vi "Traverse_Control_Ch_Names.vi"(1 "Traverse line":T1 {"Row Duration (mins)" format="%#.1f"; "Row No" min=0; "Trace Gas Concentration (%)" min=0.0 format="%#.2f"; "Emission Rate (l/min)" format="%#.2f"; "Tunnel Speed" format="%#.2f"; "Start X" format="%#.2f"; "Start Y" format="%#.2f"; "Start Z" format="%#.2f"; "End X" format="%#.2f"; "End Y" format="%#.2f"; "End Z" format="%#.2f"; "Averaging time (min)" min=0.0 format="%#.2f"}, 2 "Mode":T4(ring)) -> (0 "Channel names":string[](array[string]))   [LabVIEW 2013]
uses:
  Traverse_cluster.ctl
  Spacing.ctl
  Controls/Multi_run_mode.ctl
  Globals/Extra_Commands_Global.vi
panel:
  # "X           Y            Z"
  # "Start"
  # "End"
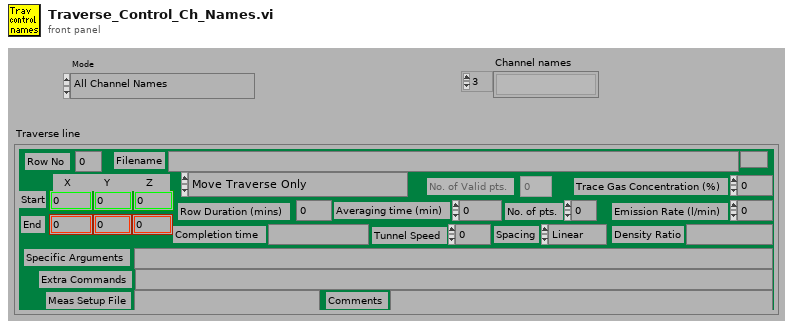
[diagram p1: front panel]
types:
  T1 = typedef "Traverse_cluster.ctl" = cluster{"Start X":dbl, "Start Y":dbl, "Start Z":dbl, "End X":dbl, "End Y":dbl, "End Z":dbl, "No. of pts.":i32, "Spacing":T2, "Filename":path, "Tunnel Speed":dbl, "Averaging time (min)":dbl, "Extra Commands":string, "Specific Arguments":string, "Emission Rate (l/min)":dbl, "Trace Gas Concentration (%)":dbl, "Density Ratio":string, "Comments":string, "Row No":i32, "Row Type Selector":T3, "Completion time":string, "Row Duration (mins)":dbl, "No. of Valid pts.":i32, "Meas Setup File":string}
  T2 = typedef "Spacing.ctl" = enum16{"Linear", "Log", "Gauss", "Specified", "N/A"}
  T3 = typedef "Multi_run_mode.ctl" = enum16{"Move Traverse Only", "Set Tunnel Speed Only", "Set Source Only", "Set Measurement Conditions", "Single Measurement", "Vertical Profile", "Lateral Profile", "Longitudinal Profile", "Explore Volume", "Multi-Axis Profile", "Auto Calibrate", "Meas Fast FID Bkgnd", "Check Beam Power", "Scanning Valve Measurement", "Run VI Named:", "Set ADAM Ch", "Wait (minutes)", "Send Message", "Synchronize With:", "Fall Back to this Row", "Turn Off Row Repeating", "Blank Row", "Traverse 3D Volume"}
  T4 = enum16{"All Channel Names", "Valid Channel Names"}
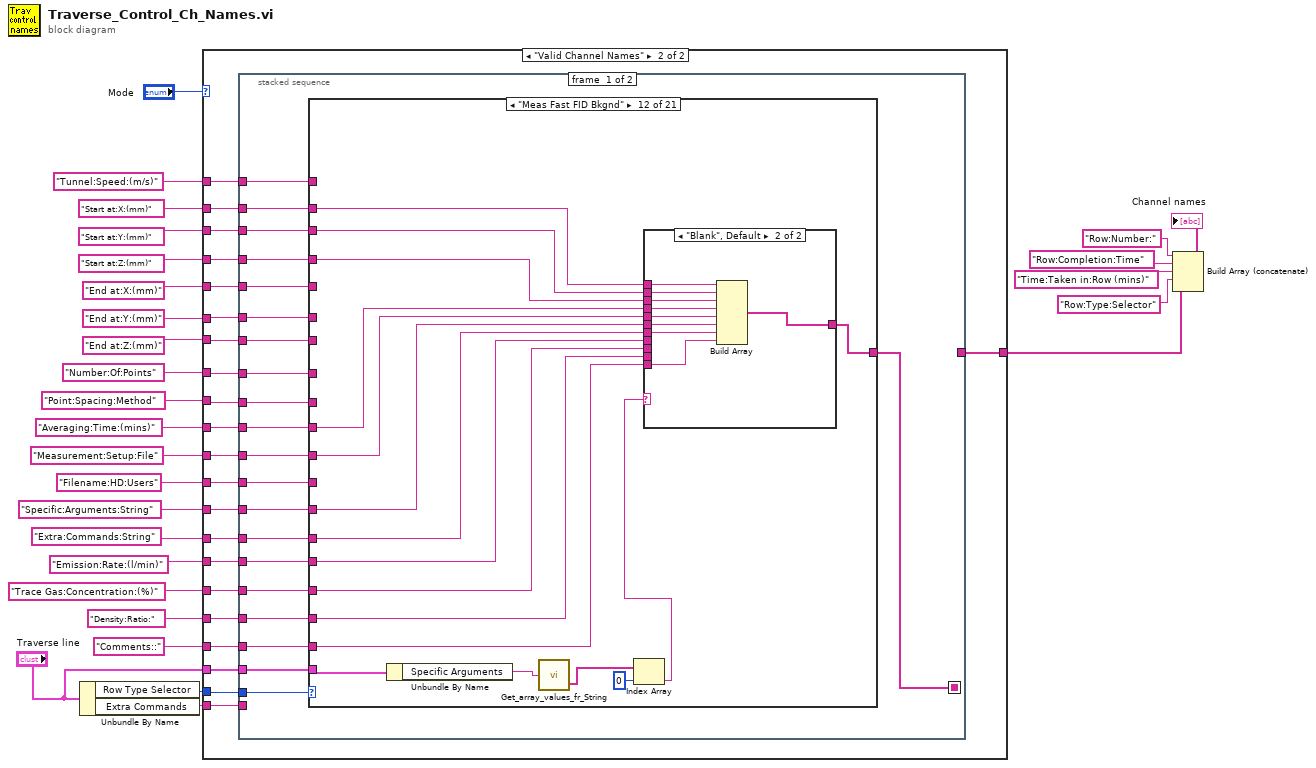
[diagram p0: block diagram]
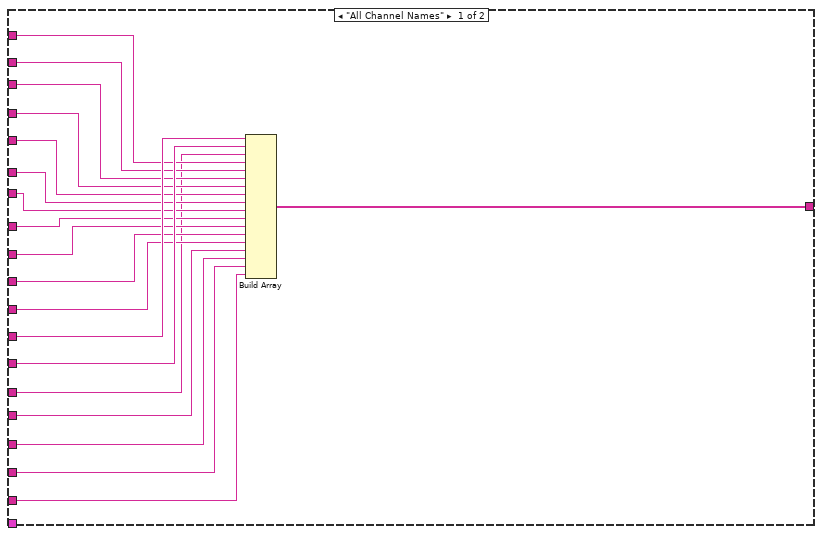
[diagram p2: hidden frame]
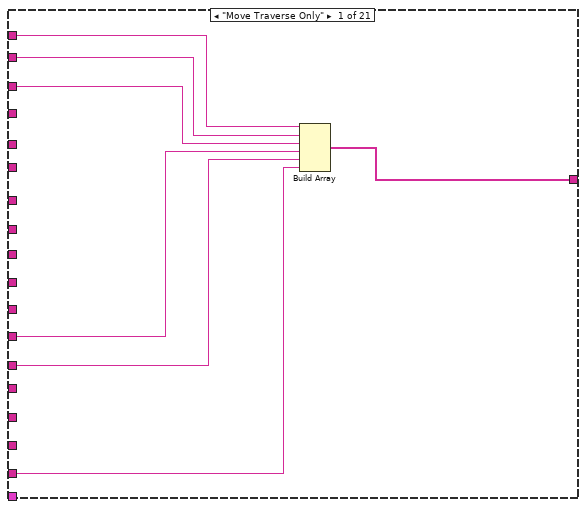
[diagram p3: hidden frame]
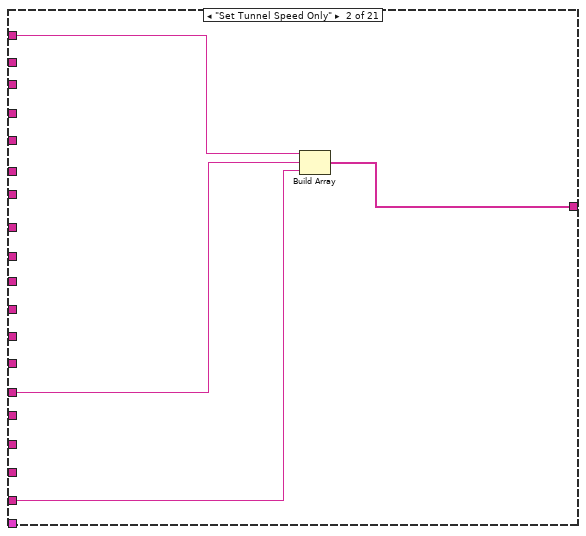
[diagram p4: hidden frame]
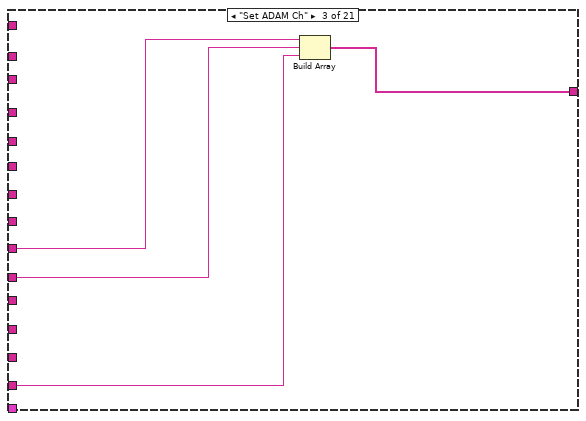
[diagram p5: hidden frame]
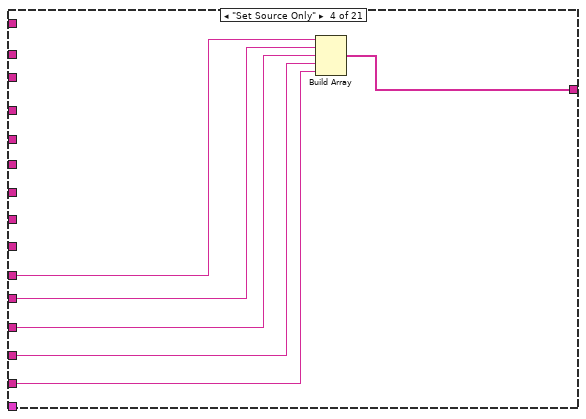
[diagram p6: hidden frame]
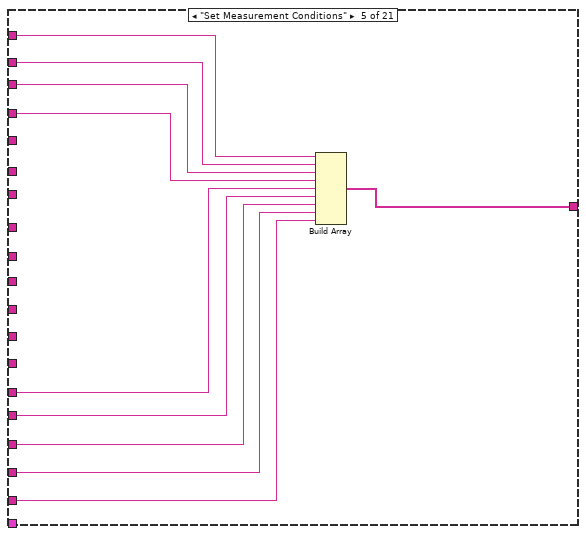
[diagram p7: hidden frame]
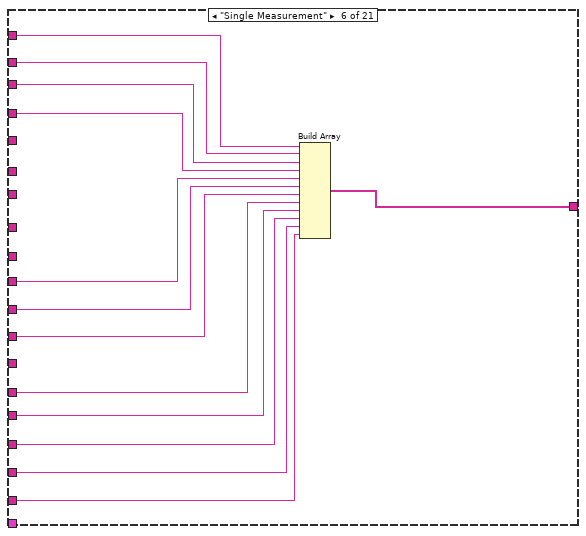
[diagram p8: hidden frame]
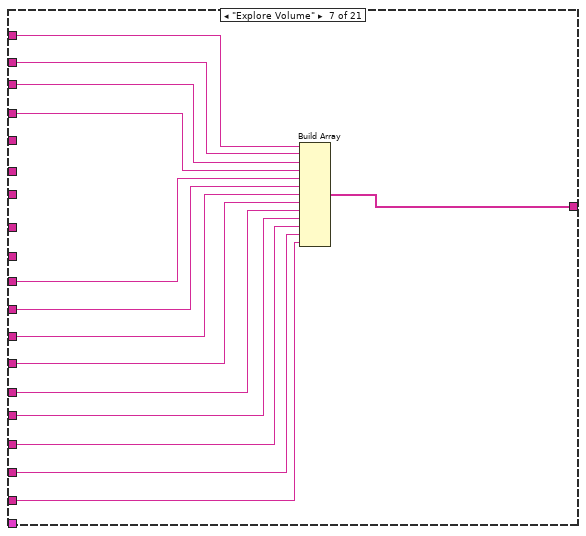
[diagram p9: hidden frame]
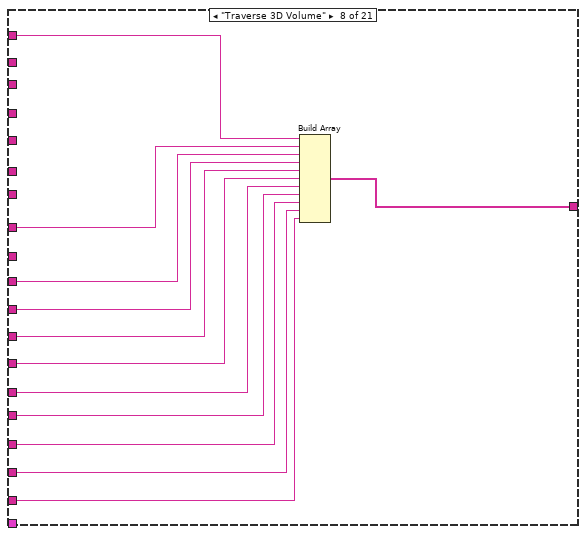
[diagram p10: hidden frame]
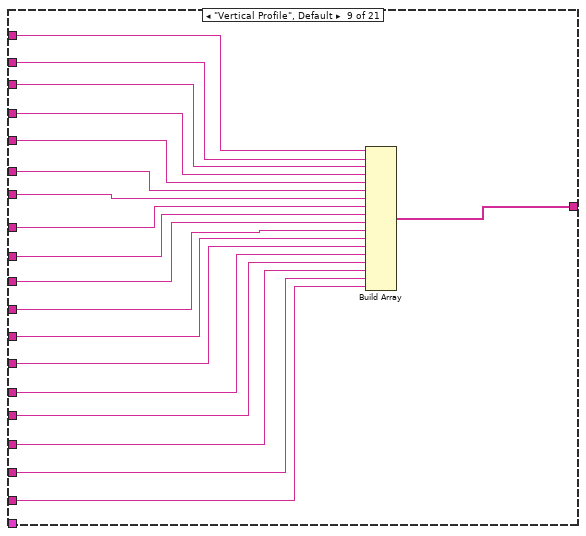
[diagram p11: hidden frame]
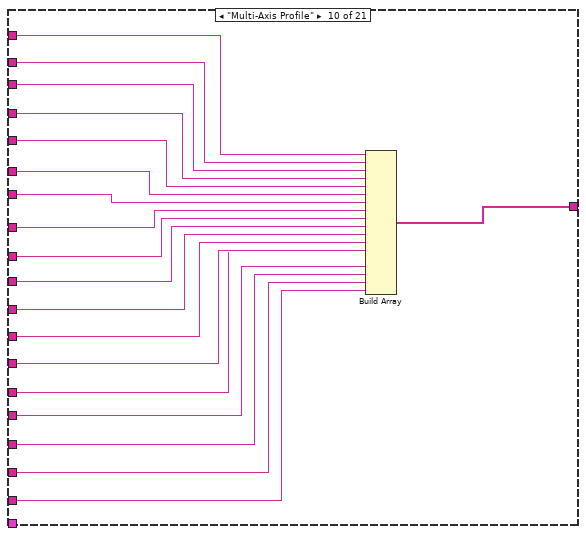
[diagram p12: hidden frame]
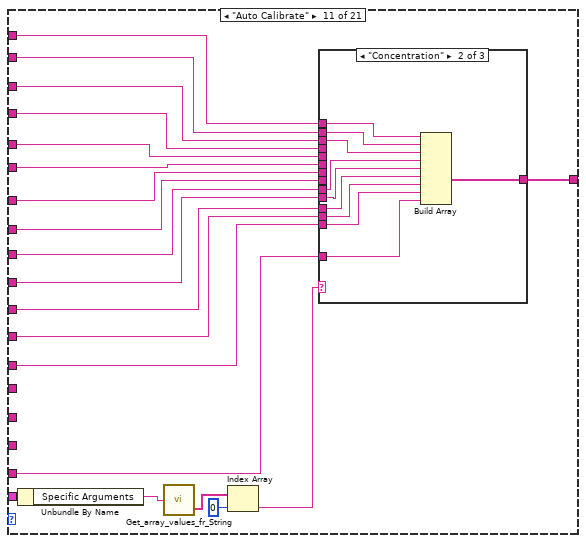
[diagram p13: hidden frame]
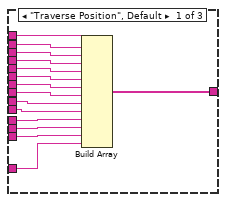
[diagram p14: hidden frame]
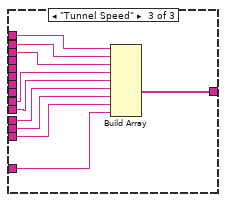
[diagram p15: hidden frame]
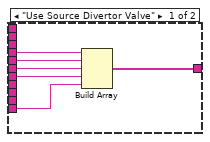
[diagram p16: hidden frame]
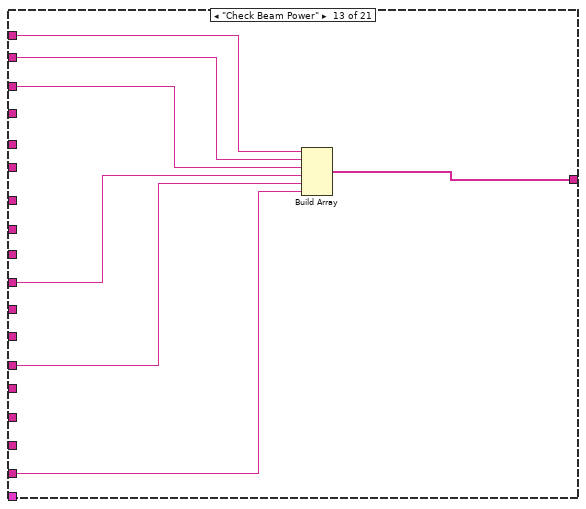
[diagram p17: hidden frame]
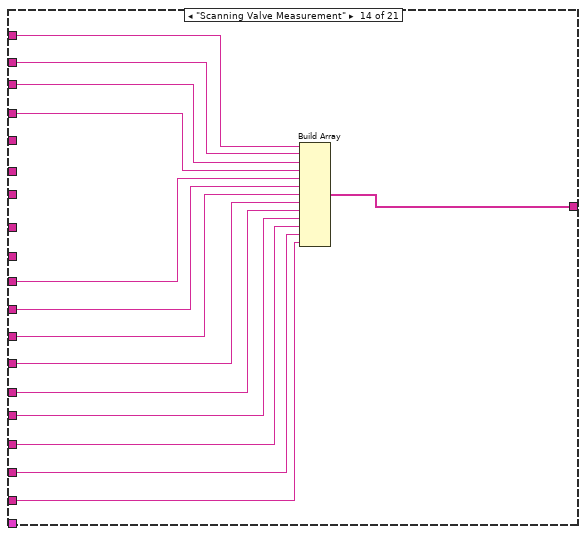
[diagram p18: hidden frame]
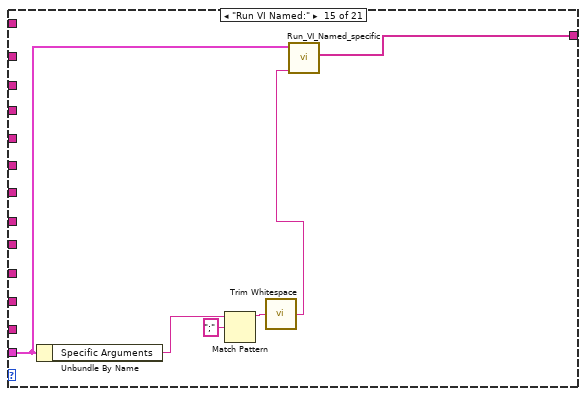
[diagram p19: hidden frame]
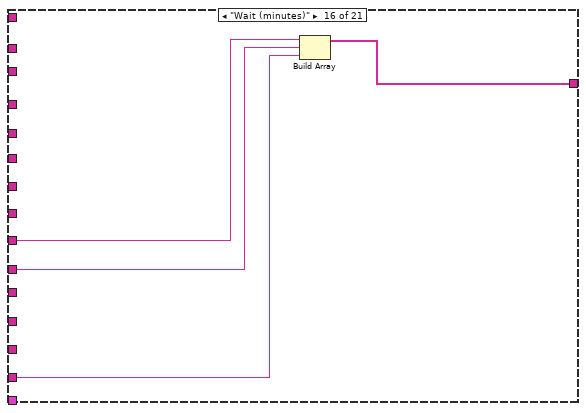
[diagram p20: hidden frame]
diagram:
  n1 = Unbundle By Name("Traverse line") -> ("Row Type Selector"=w10:T3, "Extra Commands"=w1:string)
  n2 = case shown="\"Valid Channel Names\"" "Mode" {
    tunnel: "Tunnel:Speed:(m/s)" ("Label for value") -> [w44 w68]
    tunnel: "Start at:X:(mm)" ("Label for value") -> [w43 w67]
    tunnel: "Start at:Y:(mm)" ("Label for value") -> [w42 w66]
    tunnel: "Start at:Z:(mm)" ("Label for value") -> [w41 w65]
    tunnel: "End at:X:(mm)" ("Label for value") -> [w40 w55]
    tunnel: "End at:Y:(mm)" ("Label for value") -> [w39 w54]
    tunnel: "End at:Z:(mm)" ("Label for value") -> [w38 w53]
    tunnel: "Number:Of:Points" ("Label for value") -> [w37 w52]
    tunnel: "Point:Spacing:Method" ("Label for value") -> [w36 w51]
    tunnel: "Averaging:Time:(mins)" ("Label for value") -> [w35 w57]
    tunnel: "Filename:HD:Users" ("Label for value") -> [w46 w64]
    tunnel: "Specific:Arguments:String" ("Label for value") -> [w45 w56]
    tunnel: "Extra:Commands:String" ("Label for value") -> [w29 w63]
    tunnel: "Emission:Rate:(l/min)" ("Label for value") -> [w34 w62]
    tunnel: "Trace Gas:Concentration:(%)" ("Label for value") -> [w33 w61]
    tunnel: "Density:Ratio:" ("Label for value") -> [w32 w60]
    tunnel: "Comments::" ("Label for value") -> [w31 w59]
    tunnel: w10 -> [_ w69]
    tunnel: [w47 w58] -> w6
    tunnel: "Traverse line" -> [_ w50]
    tunnel: "Measurement:Setup:File" ("Label for value") -> [w30 w49]
    tunnel: w1 -> [_ w48]
    frame "All Channel Names" {
      n3 = Build Array(w46, w45, w29, w44, w43, w42, w41, w40, w39, w38, w37, w36, w35, w30, w34, w33, w32, w31) -> (w47:string[])
    }
    frame "Valid Channel Names" {
      n4 = stacked-sequence {
        seq-local: [w70 _] -> [_ w344]
        tunnel: w69 -> [w90 _]
        tunnel: w68 -> [w89 w342]
        tunnel: w67 -> [w88 w341]
        tunnel: w66 -> [w87 w340]
        tunnel: w65 -> [w86 w339]
        tunnel: w64 -> [w85 _]
        tunnel: w63 -> [w84 _]
        tunnel: w62 -> [w83 w331]
        tunnel: w61 -> [w82 w332]
        tunnel: w60 -> [w81 w333]
        tunnel: w59 -> [w80 _]
        tunnel: [_ w345] -> w58
        tunnel: w57 -> [w79 _]
        tunnel: w56 -> [w78 _]
        tunnel: w55 -> [w77 w338]
        tunnel: w54 -> [w76 w337]
        tunnel: w53 -> [w75 w336]
        tunnel: w52 -> [w74 w335]
        tunnel: w51 -> [w73 w334]
        tunnel: w50 -> [w72 _]
        tunnel: w49 -> [w71 _]
        tunnel: w48 -> [_ w343]
        frame #0 {
          n5 = case shown="\"Meas Fast FID Bkgnd\"" w90 {
            tunnel: w89 -> [_ w100 _ _ w120 w134 w148 w150 w179 w198 _ _ _ w306 _ _ _ _ _ _ _]
            tunnel: w88 -> [w97 _ _ _ w119 w133 w147 _ w178 w197 w218 w266 w288 w305 _ _ _ _ _ _ _]
            tunnel: w87 -> [w96 _ _ _ w118 w132 w146 _ w177 w196 w217 w265 w287 w304 _ _ _ _ _ _ _]
            tunnel: w86 -> [w95 _ _ _ w117 w131 w145 _ w176 w195 w216 w264 w286 w303 _ _ _ _ _ _ _]
            tunnel: w85 -> [_ _ _ _ _ w128 w142 w158 w168 w187 w209 _ _ w300 _ _ w317 _ _ _ _]
            tunnel: w84 -> [w93 w99 w102 w110 w116 w123 w137 w153 w166 w185 w207 w268 w290 w298 _ w314 w319 _ _ _ _]
            tunnel: w83 -> [_ _ _ w109 w115 w127 w141 w157 w165 w184 _ w262 _ w297 _ _ _ _ _ _ _]
            tunnel: w82 -> [_ _ _ w108 w114 w126 w140 w156 w164 w183 _ w261 _ w296 _ _ _ _ _ _ _]
            tunnel: w81 -> [_ _ _ w107 w113 w125 w139 w155 w163 w182 _ w260 _ w295 _ _ _ _ _ _ _]
            tunnel: w80 -> [w92 w98 w104 w106 w112 w124 w138 w154 w162 w181 w206 w269 w291 w294 _ w313 w318 w322 w325 w327 w330]
            tunnel: [w94 w101 w105 w111 w121 w130 w144 w160 w175 w194 w215 w270 w292 w302 w307 w316 w321 w324 w326 w328 w329] -> w70
            tunnel: w79 -> [_ _ _ _ _ w129 w143 w159 w169 w188 w203 w263 _ w301 _ _ _ _ _ _ _]
            tunnel: w78 -> [w91 _ w103 _ _ _ w136 w152 w167 w186 w208 w267 _ w299 _ w315 w320 w323 _ _ _]
            tunnel: w77 -> [_ _ _ _ _ _ _ _ w174 w193 w214 _ _ _ _ _ _ _ _ _ _]
            tunnel: w76 -> [_ _ _ _ _ _ _ _ w173 w192 w213 _ _ _ _ _ _ _ _ _ _]
            tunnel: w75 -> [_ _ _ _ _ _ _ _ w172 w191 w212 _ _ _ _ _ _ _ _ _ _]
            tunnel: w74 -> [_ _ _ _ _ _ _ w149 w171 w190 w211 _ _ _ _ _ _ _ _ _ _]
            tunnel: w73 -> [_ _ _ _ _ _ _ _ w170 w189 w210 _ _ _ _ _ _ _ _ _ _]
            tunnel: w72 -> [_ _ _ _ _ _ _ _ _ _ w205 w255 _ _ w308 _ _ _ _ _ _]
            tunnel: w71 -> [_ _ _ _ _ w122 w135 w151 w161 w180 w204 w259 w289 w293 _ _ _ _ _ _ _]
            frame "Move Traverse Only" {
              n6 = Build Array(w97, w96, w95, w91, w93, w92) -> (w94:string[])
            }
            frame "Set Tunnel Speed Only" {
              n7 = Build Array(w100, w99, w98) -> (w101:string[])
            }
            frame "Set ADAM Ch" {
              n8 = Build Array(w103, w102, w104) -> (w105:string[])
            }
            frame "Set Source Only" {
              n9 = Build Array(w110, w109, w108, w107, w106) -> (w111:string[])
            }
            frame "Set Measurement Conditions" {
              n10 = Build Array(w120, w119, w118, w117, w116, w115, w114, w113, w112) -> (w121:string[])
            }
            frame "Single Measurement" {
              n11 = Build Array(w134, w133, w132, w131, w129, w122, w128, w123, w127, w126, w125, w124) -> (w130:string[])
            }
            frame "Explore Volume" {
              n12 = Build Array(w148, w147, w146, w145, w143, w135, w142, w136, w137, w141, w140, w139, w138) -> (w144:string[])
            }
            frame "Traverse 3D Volume" {
              n13 = Build Array(w150, w149, w159, w151, w158, w152, w153, w157, w156, w155, w154) -> (w160:string[])
            }
            frame "Vertical Profile", Default {
              n14 = Build Array(w179, w178, w177, w176, w174, w173, w172, w171, w170, w169, w161, w168, w167, w166, w165, w164, w163, w162) -> (w175:string[])
            }
            frame "Multi-Axis Profile" {
              n15 = Build Array(w198, w197, w196, w195, w193, w192, w191, w190, w189, w188, w180, w187, w186, w185, w184, w183, w182, w181) -> (w194:string[])
            }
            frame "Auto Calibrate" {
              n16 = Unbundle By Name(w205) -> ("Specific Arguments"=w202:string)
              n17 = call "Get_array_values_fr_String.vi"("String Value"=w202) -> ("String array"=w200:string[])  [unwired: 1 out]
              n18 = Index Array(array=w200, index=0 ("Index")) -> (element=w199:string)
              n19 = case shown="\"Concentration\"" w199 {
                tunnel: w218 -> [w233 w243 w253]
                tunnel: w217 -> [w232 w242 w252]
                tunnel: w216 -> [w231 w241 w251]
                tunnel: [w230 w240 w250] -> w215
                tunnel: w214 -> [w229 _ _]
                tunnel: w213 -> [w228 _ _]
                tunnel: w212 -> [w227 _ _]
                tunnel: w211 -> [w226 _ _]
                tunnel: w210 -> [w225 _ _]
                tunnel: w209 -> [w224 w239 w249]
                tunnel: w208 -> [w223 w238 w248]
                tunnel: w207 -> [w222 w237 w247]
                tunnel: w206 -> [w221 w236 w246]
                tunnel: w204 -> [w220 w235 w245]
                tunnel: w203 -> [w219 w234 w244]
                frame "Traverse Position", Default {
                  n20 = Build Array(w233, w232, w231, w229, w228, w227, w226, w225, w219, w220, w224, w223, w222, w221) -> (w230:string[])
                }
                frame "Concentration" {
                  n21 = Build Array(w243, w242, w241, w234, w235, w239, w238, w237, w236) -> (w240:string[])
                }
                frame "Tunnel Speed" {
                  n22 = Build Array(w253, w252, w251, w244, w245, w249, w248, w247, w246) -> (w250:string[])
                }
              }
            }
            frame "Meas Fast FID Bkgnd" {
              n23 = Unbundle By Name(w255) -> ("Specific Arguments"=w257:string)
              n24 = call "Get_array_values_fr_String.vi"("String Value"=w257) -> ("String array"=w256:string[])  [unwired: 1 out]
              n25 = Index Array(array=w256, index=0) -> (element=w254:string)
              n26 = case shown="\"Blank\", Default" w254 {
                tunnel: [w276 w285] -> w270
                tunnel: w269 -> [w275 w284]
                tunnel: w268 -> [w274 w283]
                tunnel: w267 -> [w273 w282]
                tunnel: w266 -> [_ w278]
                tunnel: w265 -> [_ w277]
                tunnel: w264 -> [_ w281]
                tunnel: w263 -> [w272 w280]
                tunnel: w262 -> [_ _]
                tunnel: w261 -> [_ _]
                tunnel: w260 -> [_ _]
                tunnel: w259 -> [w271 w279]
                frame "Use Source Divertor Valve" {
                  n27 = Build Array(w272, w271, w273, w274, w275) -> (w276:string[])
                }
                frame "Blank", Default {
                  n28 = Build Array(w278, w277, w281, w280, w279, w282, w283, w284) -> (w285:string[])
                }
              }
            }
            frame "Check Beam Power" {
              n29 = Build Array(w288, w287, w286, w289, w290, w291) -> (w292:string[])
            }
            frame "Scanning Valve Measurement" {
              n30 = Build Array(w306, w305, w304, w303, w301, w293, w300, w299, w298, w297, w296, w295, w294) -> (w302:string[])
            }
            frame "Run VI Named:" {
              n31 = Unbundle By Name(w308) -> ("Specific Arguments"=w310:string)
              n32 = Match Pattern(string=w310, regular expression=";") -> (before substring=w312:string)  [unwired: 4 out]
              n33 = call <vilib>:"Trim Whitespace.vi"("string"=w312) -> ("trimmed string"=w309:string)  [unwired: 1 in]
              n34 = call "Run_VI_Named_specific.vi"("Run VI Named String"=w309, "Multi Run Row"=w308) -> ("Channel Names"=w307:string[])  [unwired: 9 out]
            }
            frame "Wait (minutes)" {
              n35 = Build Array(w315, w314, w313) -> (w316:string[])
            }
            frame "Send Message" {
              n36 = Build Array(w317, w320, w319, w318) -> (w321:string[])
            }
            frame "Synchronize With:" {
              n37 = Build Array(w323, w322) -> (w324:string[])
            }
            frame "Fall Back to this Row" {
              n38 = Build Array(w325) -> (w326:string[])
            }
            frame "Blank Row" {
              n39 = Build Array(w327) -> (w328:string[])
            }
            frame "Turn Off Row Repeating" {
              n40 = Build Array(w330) -> (w329:string[])
            }
          }
        }
        frame #1 {
          n41 = Empty String/Path?(string/path=w343) -> (empty?=w346:bool)
          n42 = case shown="True" w346 {
            tunnel: [w347 w405] -> w345
            tunnel: w344 -> [w349 w405]
            tunnel: w343 -> [w353 _]
            tunnel: w342 -> [w360 _]
            tunnel: w341 -> [w372 _]
            tunnel: w340 -> [w371 _]
            tunnel: w339 -> [w370 _]
            tunnel: w338 -> [w369 _]
            tunnel: w337 -> [w368 _]
            tunnel: w336 -> [w367 _]
            tunnel: w335 -> [w366 _]
            tunnel: w334 -> [w365 _]
            tunnel: w333 -> [w358 _]
            tunnel: w332 -> [w357 _]
            tunnel: w331 -> [w356 _]
            frame False {
              n43 = global read "Extra_Commands_Global.vi" "Skip Traverse Position Demand"() -> (w373:string)
              n44 = global read "Extra_Commands_Global.vi" "Skip Tunnel Speed Demand"() -> (w362:string)
              n45 = Match Pattern(string=w353, regular expression=w373) -> (offset past match=w374:i32)  [unwired: 4 out]
              n46 = global read "Extra_Commands_Global.vi" "Skip Source Demand"() -> (w352:string)
              n47 = Match Pattern(string=w353, regular expression=w362) -> (offset past match=w363:i32)  [unwired: 4 out]
              n48 = Greater Than 0?(x=w374) -> (x > 0?=w364:bool)
              n49 = case shown="True" w364 {
                tunnel: w372 -> [_ w404]
                tunnel: w371 -> [_ w403]
                tunnel: w370 -> [_ w402]
                tunnel: w369 -> [_ w401]
                tunnel: w368 -> [_ w400]
                tunnel: w367 -> [_ w399]
                tunnel: w366 -> [_ w398]
                tunnel: w365 -> [_ w397]
                tunnel: [string[] [] w396] -> w359
                frame False {
                }
                frame True {
                  n50 = Build Array(w404, w403, w402, w401, w400, w399, w398, w397) -> (w396:string[])
                }
              }
              n51 = Greater Than 0?(x=w363) -> (x > 0?=w361:bool)
              n52 = case shown="True" w361 {
                tunnel: w360 -> [_ w394]
                tunnel: w359 -> [w391 w393]
                tunnel: [w391 w392] -> w355
                frame False {
                }
                frame True {
                  n53 = Build Array (concatenate)(w394, w393) -> (w392:string[])
                }
              }
              n54 = Match Pattern(string=w353, regular expression=w352) -> (offset past match=w354:i32)  [unwired: 4 out]
              n55 = Greater Than 0?(x=w354) -> (x > 0?=w351:bool)
              n56 = case shown="False" w351 {
                tunnel: w356 -> [_ w390]
                tunnel: w357 -> [_ w389]
                tunnel: w358 -> [_ w388]
                tunnel: [w385 w387] -> w350
                tunnel: w355 -> [w385 w386]
                frame False {
                }
                frame True {
                  n57 = Build Array (concatenate)(w386, w390, w389, w388) -> (w387:string[])
                }
              }
              n58 = for {
                shift-right: [w375] -> w347
                shift-left: string[] [] -> [w377]
                tunnel: w350 -> [w380]
                tunnel: w349 -> [w376] mode=indexing
                n59 = Search 1D Array(1D array=w380, element=w376) -> (index of element=w379:i32)  [unwired: 1 out]
                n60 = Less Than 0?(x=w379) -> (x < 0?=w378:bool)
                n61 = case shown="True" w378 {
                  tunnel: w377 -> [w381 w384]
                  tunnel: w376 -> [_ w383]
                  tunnel: [w381 w382] -> w375
                  frame False {
                  }
                  frame True {
                    n62 = Build Array (concatenate)(w384, w383) -> (w382:string[])
                  }
                }
              }
            }
            frame True {
            }
          }
        }
      }
    }
  }
  n63 = Build Array (concatenate)("Row:Number:" ("Label for value"), "Row:Completion:Time" ("Label for value"), "Time:Taken in:Row (mins)" ("Label for value"), "Row:Type:Selector" ("Label for value"), w6) -> (→"Channel names":string[])
